vi "No Modal for Dev.vi"   [LabVIEW 2020, in "Conditum-Tools.lvlib"]
doc: "If the VI is Modal and the \"Conditum_Dev\" conditional symbol == True then the FP behavior is changed to Floating for debuggability."
uses:
  Conditum-Tools.lvlib
types:
  T1 = enum32{"Invalid", "Default", "Floating", "Floating/Auto-Hide", "Modal"}
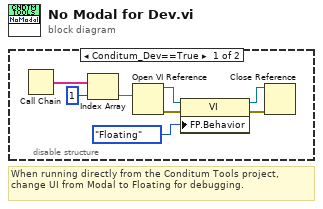
[diagram p0: block diagram]
diagram:
  # "When running directly from the Conditum Tools project, change UI from Modal to Floating for debugging."
  n1 = disable-structure shown="Conditum_Dev==True" {
    frame condition #0 (active) {
      n2 = Call Chain() -> (call chain=w8:string[])
      n3 = Index Array(array=w8, index=1) -> (element=w7:string)
      n4 = Open VI Reference(vi path=w7) -> (vi reference=w1:refnum<vi>, error out=w2:errorcluster)  [unwired: 5 in]
      n5 = property class="VI"(reference=w1, error in=w2, "FP.Behavior"=T1."Floating" ("Front Panel Window:Behavior")) -> (reference out=w5:refnum<vi>, error out=w6:errorcluster)
      n6 = Close Reference(reference=w5, error in (no error)=w6) -> ()  [unwired: 1 out]
    }
    frame condition #1 {
    }
  }
